vi "exp4.vi"() -> ()   [LabVIEW 2020]
doc: "This example demonstrates the implementation of Equalization in an QAM Modulation Demodulation System"
uses:
  <vilib>/addons/Modulation/Digital/General/MT Generate Bits (Galois, PN Order).vi
  <vilib>/addons/Modulation/Analog/support/mod_Set Error Source.vi
  <vilib>/addons/Modulation/Digital/Support/Common/Validators/mod_Generate Bits Validate.vi
  <vilib>/addons/Modulation/Digital/Support/Common/Validators/mod_AWGN Validate.vi
  <vilib>/addons/Modulation/Digital/Impairments/subVIs/mod_createSeeds.vi
  <vilib>/addons/Modulation/Digital/Support/Common/Validators/mod_Validate Samples Per Symbol.vi
  <vilib>/addons/Modulation/Analog/support/Validators/mod_Validate Complex Waveform.vi
  <vilib>/addons/Modulation/Analog/support/Validators/mod_WFErrorHandler.vi
  <vilib>/measure/masml.llb/ma_sml_Interpolation by Zero Insert (complex input).vi
  <vilib>/addons/Modulation/Digital/General/MT Generate QAM System Parameters(M).vi
  <vilib>/addons/Modulation/Digital/Support/Common/Validators/mod_Generate Filter Coefficients Validate.vi
  <vilib>/addons/Modulation/Digital/General/subVIs/mod_Generate Filter Coefficients.vi
  <vilib>/addons/Modulation/Digital/General/subVIs/mod_Generate Bits PN Sequence.vi
  <vilib>/Analysis/1siggen.llb/Gaussian White Noise (obs 90).vi
  <vilib>/addons/Modulation/Digital/General/MT Apply Matched Filter (Generic).vi
  <vilib>/addons/Modulation/Digital/General/MT Align to Ideal Symbols (Generic).vi
  <vilib>/addons/Modulation/Digital/Demodulation/MT Calculate BER After Trigger (PN Sequence).vi
  <vilib>/addons/Modulation/niDMT.lvlib
  <vilib>/Analysis/NI_AALBase.lvlib
  <vilib>/measure/NI_MAPro.lvlib
panel:
  out "Error Out":errorcluster
  in  "Error In":errorcluster
  in  "Reset?":bool
  out "Recovered":i8[](array[numeric])
  out "Message":i8[](array[numeric])
  in  "Equalizer length \n(symbols)":i32=48
  in  "PN Sequence Order":i32=26
  in  "Channel Filter Length\n(symbols)":i32=8
  out "BER Trigger Found Index (Bits)":u32
  out "Optimal Offset (Samples)":dbl format="%.4f"
  in  "Seed In":i32=-1
  out "Modulation Error Ratio (dB)":dbl format="%.2f"
  in  "Training Length\n(symbols)":i32=500
  in  "Channel Filter":T1(ring)=enum."Low-pass"
  out "BER":dbl format="%.4f"
  in  "Eb/N0 (10 dB)":dbl=50.0 format="%.2f"
  in  "Tab Control":T2(tab)=enum."RX Constellation (post equ)"
  in  "autoscale Tx":bool
  out "Constellation Graph (pre equ)":T3(graph)
  in  "Reset action":string="The example VI performs the following actions depending on the\nvalue of the boolean controls Reset? and Retrain Equalizer? :\n\n1. Reset?=TRUE: Reset all internal VIs,initialize equalizer coefficient array to equal the time-delayed dirac delta response {0 0 0... 1 ...0 0 0}, and feed training bits for equalization.\n\n2. Reset?=FALSE, Retrain Equalizer?=TRUE: Reset all receiver side VIs only,continue training the equalizer, and use final equalizer coefficient array from output of previous iteration as initial conditions for equalizer in current iteration\n\n3. Reset?=FALSE, Retrain Equalizer?=FALSE: Continue modulation, demodulation and equalization from previous iteration, while performing equalization in decision directed mode. This simulates the steady-state performance of the system once the equalizer error has fallen below a tolerance level."
  in  "autoscale Rx":bool
  out "Constellation Graph (post equ)":T3(graph)
  out "MER History":dbl(graph)=58.81121522824558
  out "LMS Error":dbl[](graph)
  out "Magnitude":dbl[][](graph)
  in  "Feedforward Equalizer (LMS)":T4={"Taps per Symbol"=1, "Delta (training)"=0.01, "Delta (steady state)"=0.01} {"Delta (steady state)" format="%#_6p"; "Delta (training)" format="%#_6p"}
  in  "Pulse Shaping Filter":T5(ring)=enum."Root Raised Cos"
  in  "Retrain\nEqualizer?":bool=TRUE
  in  "M-QAM Symbols":i32=1500
  in  "M-QAM":i32=256
  in  "Samples Per Symbol":i32=6
  in  "stop":bool
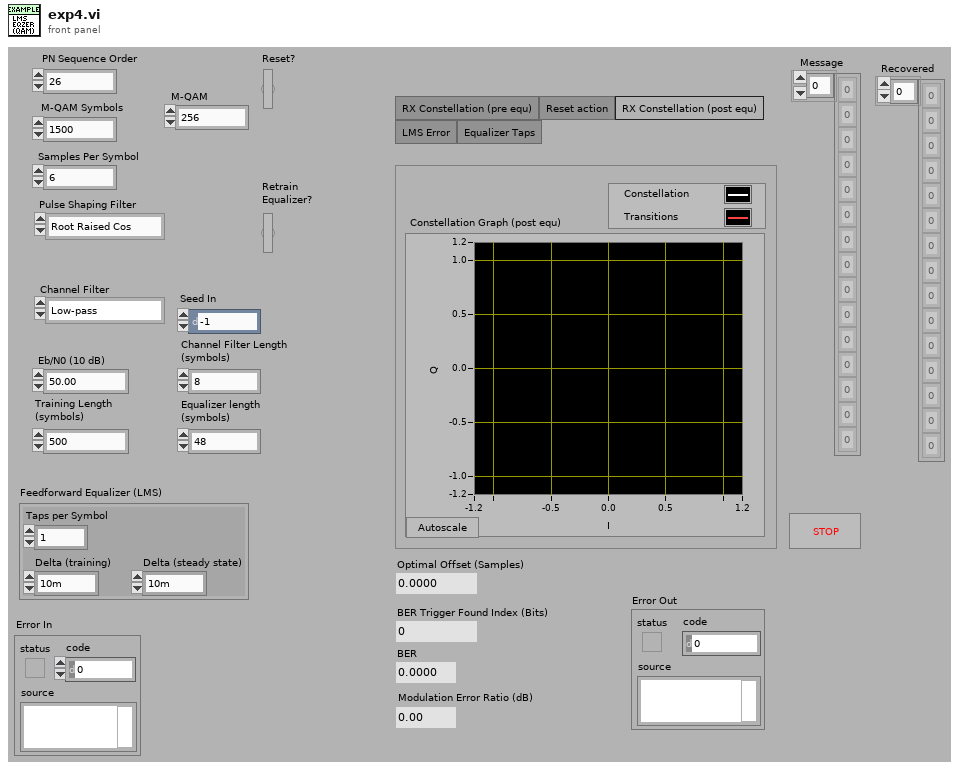
[diagram p1: front panel]
types:
  T1 = enum16{"Impulse", "Low-pass", "Custom filter", "Custom Filter-II"}
  T2 = enum32{"RX Constellation (pre equ)", "Reset action", "RX Constellation (post equ)", "LMS Error", "Equalizer Taps"}
  T3 = cluster{"Decimated Array":dbl[], "Decimated Array":dbl[]}[]
  T4 = cluster{"Taps per Symbol":i32, "Delta (training)":dbl, "Delta (steady state)":dbl}
  T5 = enum16{"none", "Raised Cosine", "Root Raised Cos", "Gaussian"}
  T6 = enum32{"None", "Hanning", "Hamming", "Triangular", "Blackman", "Exact Blackman", "Blackman-Harris", "Kaiser-Bessel", "Flat Top"}
  T7 = enum32{"Lowpass", "Highpass", "Bandpass", "Bandstop"}
  T8 = cluster{"start index (symbols)":i32, "width (symbols) (-1: all)":i32}
  T9 = cluster{"samples per symbol (16)":i32, "symbol map":cdb[]}
  T10 = typedef "niAMT.lvlib/Complex Data Waveform.ctl" = cluster{"t0":dbl, "dt":dbl, "Y":cdb[]}
  T11 = cluster{"constellation":dbl[], "oversampled data":dbl[]}[]
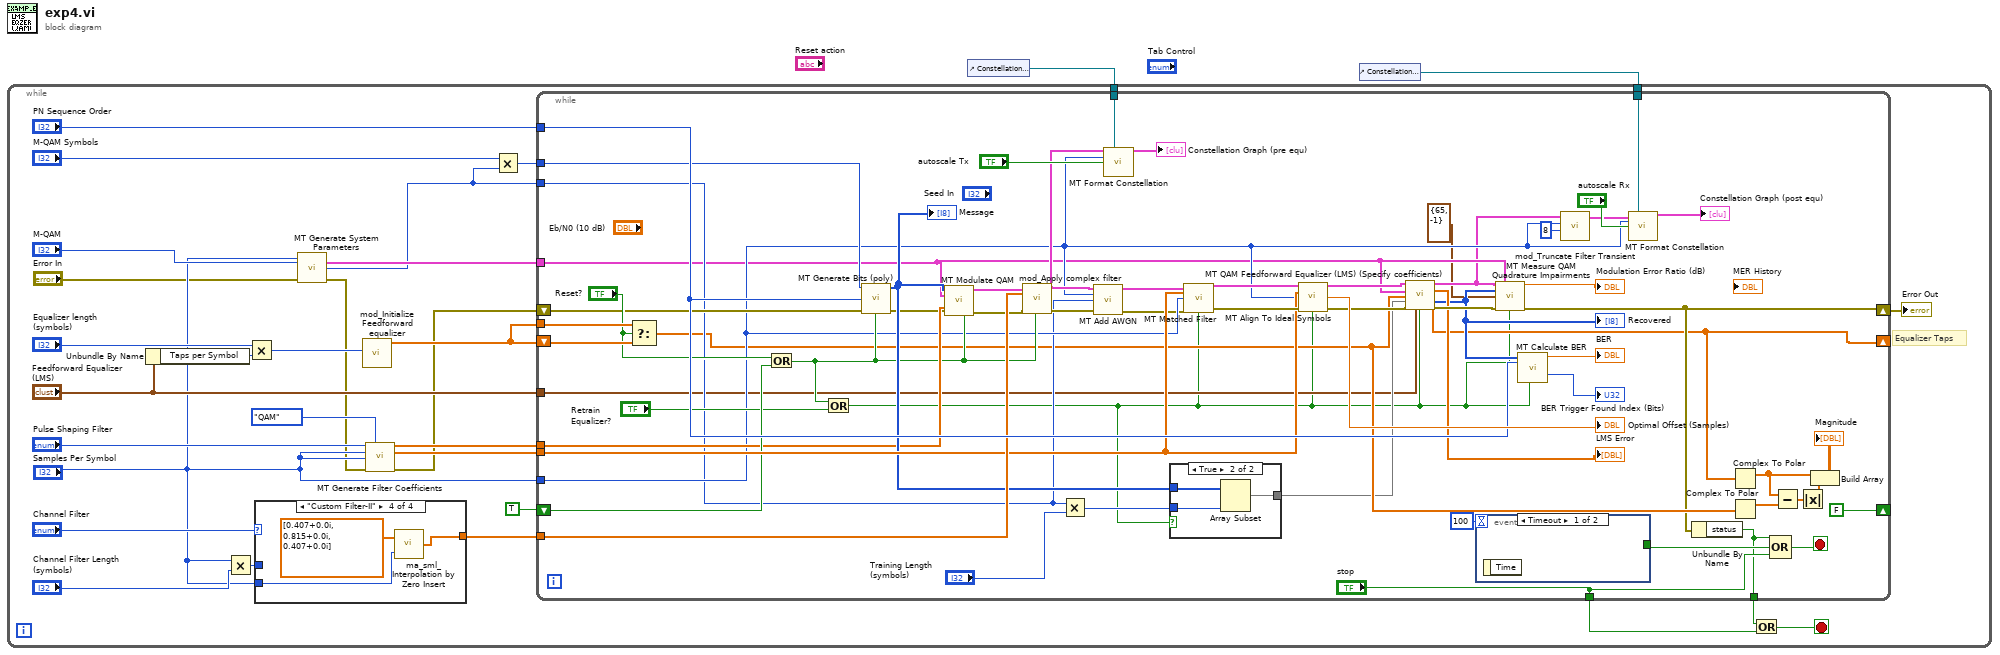
[diagram p0: block diagram]
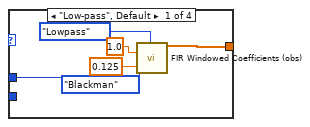
[diagram p2: hidden frame]
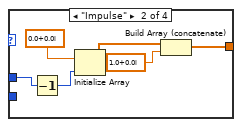
[diagram p3: hidden frame]
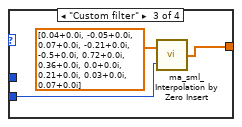
[diagram p4: hidden frame]
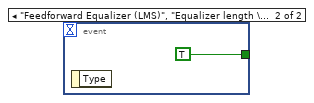
[diagram p6: hidden frame]
diagram:
  n1 = control-ref of="Constellation Graph (pre equ)"() -> (w1:refnum<vi>)
  n2 = control-ref of="Constellation Graph (post equ)"() -> (w2:refnum<vi>)
  n3 = while {
    tunnel: w2 -> [w30]
    tunnel: w1 -> [w29]
    stop <- w5 stop-if-true
    # "Equalizer Taps"
    n4 = Unbundle By Name("Feedforward Equalizer (LMS)") -> ("Taps per Symbol"=w32:i32)
    n5 = Multiply(x="Samples Per Symbol", y="Channel Filter Length\n(symbols)") -> (x*y=w26:i32)
    n6 = Multiply(x="Equalizer length \n(symbols)", y=w32) -> (x*y=w10:i32)
    n7 = case shown="\"Custom Filter-II\"" "Channel Filter" {
      tunnel: [w34 w40 w46 w49] -> w22
      tunnel: w26 -> [w33 w39 _ _]
      tunnel: "Samples Per Symbol" -> [_ _ w45 w48]
      frame "Low-pass", Default {
        n8 = call <vilib>:"FIR Windowed Coefficients (obs).vi"("filter type"=T7."Lowpass", "sampling freq: fs"=1.0, "taps"=w33, "window"=T6."Blackman", "low cutoff freq: fl"=0.125) -> ("FIR Windowed Coefficients"=w34:dbl[])  [unwired: 2 in, 8 out]
      }
      frame "Impulse" {
        n9 = Decrement(x=w39) -> (x-1=w43:i32)
        n10 = Initialize Array(cdb 0.0+0.0i ("Element Data"), w43) -> (w42:cdb[])
        n11 = Build Array (concatenate)(w42, cdb 1.0+0.0i ("Element Data")) -> (w40:cdb[])
      }
      frame "Custom filter" {
        n12 = call-poly <vilib>:"ma_sml_Interpolation by Zero Insert.vi"("L"=w45, "x"=cdb[] [0.04+0.0i, -0.05+0.0i, 0.07+0.0i, -0.21+0.0i, -0.5+0.0i, 0.72+0.0i, 0.36+0.0i, 0.0+0.0i, 0.21+0.0i, 0.03+0.0i, 0.07+0.0i]) -> ("y"=w46:cdb[])
      }
      frame "Custom Filter-II" {
        n13 = call-poly <vilib>:"ma_sml_Interpolation by Zero Insert.vi"("L"=w48, "x"=cdb[] [0.407+0.0i, 0.815+0.0i, 0.407+0.0i]) -> ("y"=w49:cdb[])
      }
    }
    n14 = call-poly <vilib>:"MT Generate System Parameters.vi"("samples per symbol (16)"="Samples Per Symbol", "M-QAM (16)"="M-QAM", "error in (no error)"="Error In") -> ("QAM system parameters"=w21:T9, "bits per symbol"=w15:i32, "error out"=w9:errorcluster)  [unwired: 10 out]
    n15 = call <vilib>:"mod_Initialize Feedforward equalizer.vi"("tap length"=w10) -> ("equalizer taps"=w11:cdb[])  [unwired: 1 in, 13 out]
    n16 = call <vilib>:"MT Generate Filter Coefficients.vi"("pulse shaping filter (none)"="Pulse Shaping Filter", "modulation type"=enum16{"FSK", "PSK", "QAM", "MSK", "PAM", "ASK"}."QAM", "pulse shaping samples per symbol (16)"="Samples Per Symbol", "matched samples per symbol (16)"="Samples Per Symbol", "error in (no error)"=w9) -> ("pulse shaping filter coefficients"=w20:dbl[], "matched filter coefficients"=w19:dbl[], "error out"=w7:errorcluster)  [unwired: 2 in, 6 out]
    n17 = Multiply(x="M-QAM Symbols", y=w15) -> (x*y=w14:i32)
    n18 = while {
      shift-right: [w53] -> _
      shift-left: w11 -> [w93]
      tunnel: ["stop"] -> w6
      tunnel: "Feedforward Equalizer (LMS)" -> [w61]
      tunnel: w30 -> [w102]
      tunnel: w29 -> [w101]
      tunnel: "PN Sequence Order" -> [w100]
      tunnel: w15 -> [w67]
      tunnel: w22 -> [w99]
      tunnel: w21 -> [w64]
      tunnel: "Samples Per Symbol" -> [w70]
      tunnel: w20 -> [w77]
      tunnel: w19 -> [w98]
      tunnel: w14 -> [w96]
      tunnel: w11 -> [w92]
      shift-right: [FALSE] -> _
      shift-left: TRUE -> [w84]
      shift-right: [w54] -> w4
      shift-left: w7 -> [w82]
      tunnel: [w52] -> w3
      stop <- w80 stop-if-true
      n19 = Select(t=w92, s="Reset?", f=w93) -> (s? t:f=w63:cdb[])
      n20 = Or(x="Reset?", y=w84) -> (x .or. y?=w73:bool)
      n21 = Or(x=w73, y="Retrain\nEqualizer?") -> (x .or. y?=w51:bool)
      n22 = call-poly <vilib>:"MT Generate Bits (poly).vi"("total bits (128)"=w96, "PN sequence order (9)"=w100, "error in (no error)"=w82, "reset? (T)"=w73) -> ("output bit stream"=w78:i8[], "error out"=w76:errorcluster)  [unwired: 1 in, 9 out]
      "Message" <- w78
      n23 = call <vilib>:"MT Modulate QAM.vi"("input bit stream"=w78, "QAM system parameters"=w64, "pulse shaping filter coefficients"=w77, "error in (no error)"=w76, "flush buffers? (F)"=w73) -> ("output complex waveform"=w75:T10, "error out"=w74:errorcluster)  [unwired: 8 in, 1 out]
      n24 = call <vilib>:"mod_Apply complex filter.vi"("input complex waveform"=w75, "filter coefficients"=w99, "reset? (T)"=w73, "error in (no error)"=w74) -> ("output complex waveform"=w72:cluster{"t0":dbl, "dt":dbl, "Y":cdb[]}, "error out"=w71:errorcluster)  [unwired: 10 out]
      n25 = Multiply(x=w67, y="Training Length\n(symbols)") -> (x*y=w107:i32)
      n26 = call <vilib>:"MT Add AWGN.vi"("input complex waveform"=w72, "samples per symbol (16)"=w70, "bits per symbol (1)"=w67, "error in (no error)"=w71) -> ("output complex waveform"=w69:T10, "error out"=w68:errorcluster)  [unwired: 9 in, 1 out]
      n27 = call <vilib>:"MT Format Constellation.vi"("waveform"=w72, "constellation reference"=w101, "samples per symbol"=w70, "autoscale"="autoscale Tx") -> ("constellation graph"=→"Constellation Graph (pre equ)":T11)  [unwired: 1 in, 10 out]
      n28 = case shown="True" w51 {
        tunnel: w78 -> [_ w116]
        tunnel: w107 -> [_ w115]
        tunnel: [_ w114] -> w62
        frame False {
        }
        frame True {
          n29 = Array Subset(array=w116, length=w115) -> (w114:i8[])  [unwired: 1 in]
        }
      }
      n30 = call-poly <vilib>:"MT Matched Filter.vi"("input complex waveform"=w69, "matched filter coefficients"=w98, "samples per symbol (16)"=w70, "error in (no error)"=w68, "reset? (T)"=w51) -> ("output complex waveform"=w104:T10, "error out"=w105:errorcluster)  [unwired: 9 out]
      n31 = call-poly <vilib>:"MT Align To Ideal Symbols.vi"("input complex waveform"=w104, "matched filter coefficients"=w98, "samples per symbol (16)"=w70, "error in (no error)"=w105, "reset? (T)"=w51) -> ("output complex waveform"=w66:T10, "waveform alignment offset (samples)"=→"Optimal Offset (Samples)":dbl, "error out"=w65:errorcluster)  [unwired: 8 out]
      n32 = call <vilib>:"MT QAM Feedforward Equalizer (LMS) (Specify coefficients).vi"("input complex waveform"=w66, "QAM system parameters"=w64, "equalizer coefficients in"=w63, "training bits"=w62, "error in (no error)"=w65, "feedforward equalizer (LMS) parameters"=w61, "reset? (T)"=w51) -> ("output complex waveform"=w57:T10, "error (V^2)"=→"LMS Error":dbl[], "equalizer coefficients out"=w53:cdb[], "output bit stream"=w58:i8[], "error out"=w60:errorcluster)  [unwired: 4 in]
      "Recovered" <- w58
      n33 = event shown="[0] Timeout" {
        selector: _ -> [_ _]
        dyn-events: _ -> [_ _]
        timeout: 100 -> [_ _]
        tunnel: [_ TRUE ("stop")] -> w81
        event Timeout {
          n34 = event-data() -> ()  [unwired: 2 out]
        }
        event "Feedforward Equalizer (LMS)", "Equalizer length \n(symbols)", "Channel Filter", "Channel Filter Length\n(symbols)", "M-QAM", "Samples Per Symbol", "Pulse Shaping Filter": Value Change {
          n35 = event-data() -> ()  [unwired: 2 out]
        }
      }
      n36 = call <vilib>:"MT Measure QAM Quadrature Impairments.vi"("recovered complex waveform"=w57, "QAM system parameters"=w64, "input bit stream"=w58, "impairment measurement window"=T8 {"start index (symbols)"=65, "width (symbols) (-1: all)"=-1}, "error in (no error)"=w60, "reset? (T)"=w51) -> ("IQ gain imbalance (dB)"=→"Modulation Error Ratio (dB)":dbl, "error out"=w54:errorcluster)  [unwired: 2 in, 6 out]
      n37 = call-poly <vilib>:"MT Calculate BER.vi"("input bit stream"=w58, "PN sequence order (9)"=w100, "reset? (T)"=w51) -> ("BER"=→"BER":dbl, "trigger found index (bits)"=→"BER Trigger Found Index (Bits)":u32)  [unwired: 3 in, 8 out]
      n38 = call <vilib>:"mod_Truncate Filter Transient.vi"("filter length (sym)"=8, "samples/symbol"=w70, "input complex waveform"=w57) -> ("output complex waveform"=w95:T10)  [unwired: 8 out]
      n39 = call <vilib>:"MT Format Constellation.vi"("waveform"=w95, "constellation reference"=w102, "samples per symbol"=w70, "autoscale"="autoscale Rx") -> ("constellation graph"=→"Constellation Graph (post equ)":T11)  [unwired: 1 in, 10 out]
      n40 = Unbundle By Name(w54) -> ("status"=w52:bool)
      n41 = Complex To Polar(r * e^(i*theta)=w53) -> (r=w89:dbl[])  [unwired: 1 out]
      n42 = Complex To Polar(r * e^(i*theta)=w63) -> (r=w88:dbl[])  [unwired: 1 out]
      n43 = Compound Arithmetic op=OR(w52, w81, "stop") -> (w80:bool)
      n44 = Subtract(x=w89, y=w88) -> (x-y=w87:dbl[])
      n45 = Absolute Value(x=w87) -> (abs(x)=w86:dbl[])
      n46 = Build Array(w89, w86) -> (→"Magnitude":dbl[][])
    }
    "Error Out" <- w4
    n47 = Or(x=w3, y=w6) -> (x .or. y?=w5:bool)
  }
